vi "lab2_usrp_packet_transceiver2.vi"() -> ()   [LabVIEW 2014]
uses:
  <vilib>/addons/Modulation/Digital/General/MT Generate Bits (Galois, PN Order).vi
  <vilib>/addons/Modulation/Analog/support/mod_Set Error Source.vi
  <vilib>/addons/Modulation/Digital/Support/Common/Validators/mod_Generate Bits Validate.vi
  var_stop.vi
  <vilib>/addons/Modulation/Digital/Support/Common/Validators/mod_Generate Filter Coefficients Validate.vi
  <vilib>/addons/Modulation/Digital/General/subVIs/mod_Generate Filter Coefficients.vi
  <vilib>/measure/maspectr.llb/FFT Power Spectrum and PSD for 1 Chan (CDB).vi
  <vilib>/addons/Modulation/Digital/General/MT Apply Matched Filter (Generic).vi
  <vilib>/addons/Modulation/Digital/General/MT Align to Ideal Symbols (Generic).vi
  <instrlib>/niUSRP/niUSRP Fetch Rx Data (CDB Cluster).vi
  <instrlib>/niUSRP/niUSRP Write Tx Data (CDB Cluster).vi
  <vilib>/addons/Modulation/Digital/General/subVIs/mod_Generate Bits PN Sequence.vi
  <vilib>/addons/Modulation/Digital/General/MT Apply Pulse Shaping Filter (Generic).vi
  <vilib>/addons/Modulation/niDMT.lvlib
  <vilib>/measure/NI_MAPro.lvlib
panel:
  out "ber":dbl
  out "received bits":i32
  out "error bits":i32
  in  "random bits":i8[](array[numeric])
  out "found?":bool
  out "# elements in queue":i32
  out "Spectrum monitor":cluster{"f0":dbl, "df":dbl, "magnitude":dbl[]}(graph)={"f0"=-0.49993781867926873, "df"=0.00012436264146250465, "magnitude"=[]}
  out "RX Constellation Map":cdb[](graph)
  out "valid?":bool
  in  "Gray code?":bool
  in  "Modulation":enum16{"PSK", "QAM"}(ring)=enum."QAM"
  out "Rx String":string
  out "packet len":u32
  in  "Send":bool
  in  "filter length (symbols)":i32=8
  in  "filter parameter":dbl=0.5 format="%.2f"
  in  "pulse shaping filter (none)":T1(ring)=enum."Raised Cosine"
  in  "M-PSK (4)":i32=16 caption="M-ARY"
  in  "samples per symbol (16)":i32=4
  out "packet bits length":i32
  in  "number of samples":i64=40000
  out "RX coerced gain":dbl format="%#_6f"
  out "RX coerced carrier frequency":dbl=915000000.0 format="%#_6p"
  out "RX coerced IQ rate":dbl=4000000.0 format="%#_6p"
  in  "RX active antenna":string="RX2"
  in  "RX gain":dbl format="%#_6f"
  in  "RX device names":refnum<k15>="192.168.10.2"
  out "TX coerced gain":dbl format="%#_6f"
  out "TX coerced carrier frequency":dbl=915000000.0 format="%#_6p"
  out "coerced IQ rate":dbl=4000000.0 format="%#_6p"
  in  "TX device names":refnum<k15>="192.168.10.2"
  in  "TX gain":dbl format="%#_6f"
  in  "carrier frequency":dbl=915000000.0 format="%#_6p"
  in  "IQ rate":dbl=800000.0 format="%#_6p"
  in  "stop":bool
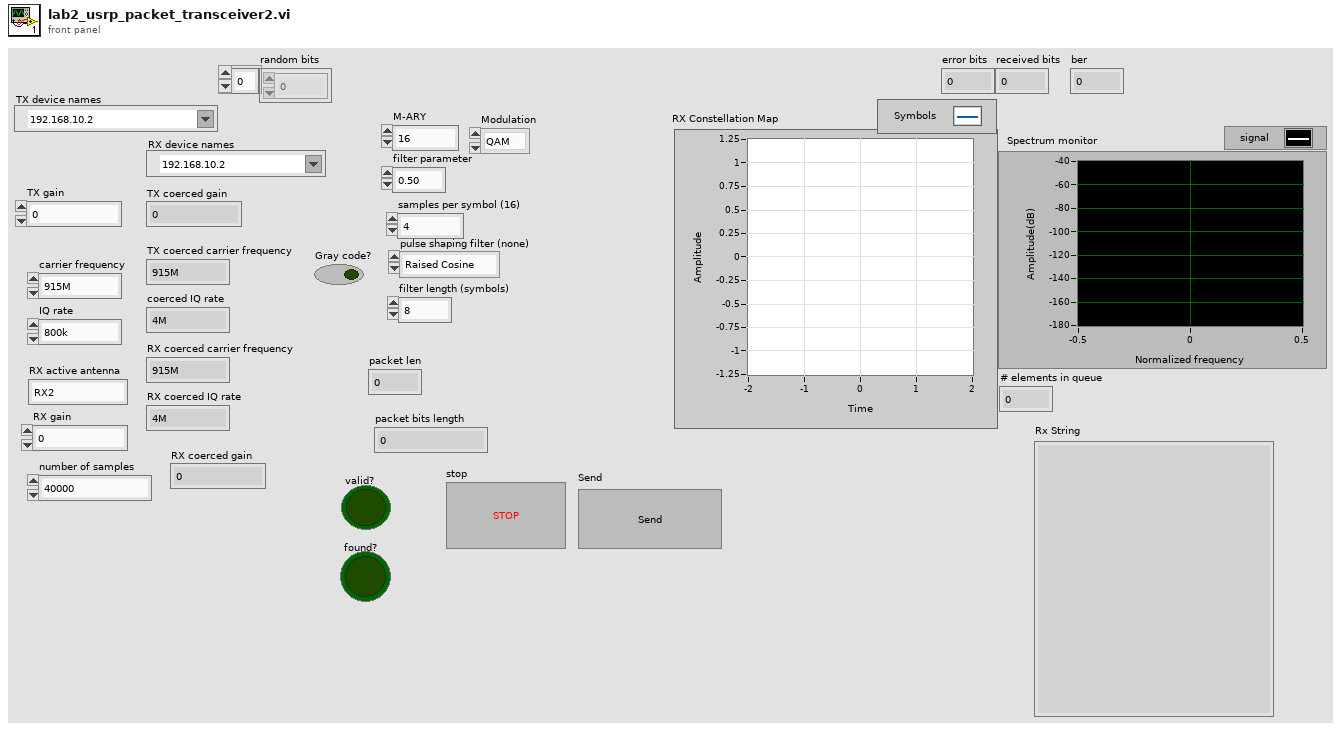
[diagram p1: front panel]
types:
  T1 = enum16{"none", "Raised Cosine", "Root Raised Cos", "Gaussian"}
  T2 = enum16{"FSK", "PSK", "QAM", "MSK", "PAM", "ASK", "CPM"}
  T3 = cluster{"samples per symbol (16)":i32, "symbol map":cdb[], "index map":u32[]}
  T4 = cluster{"samples per symbol (16)":i32, "symbol map":cdb[], i32[]}
  T5 = typedef "niAMT.lvlib/Complex Data Waveform.ctl" = cluster{"t0":dbl, "dt":dbl, "Y":cdb[]}
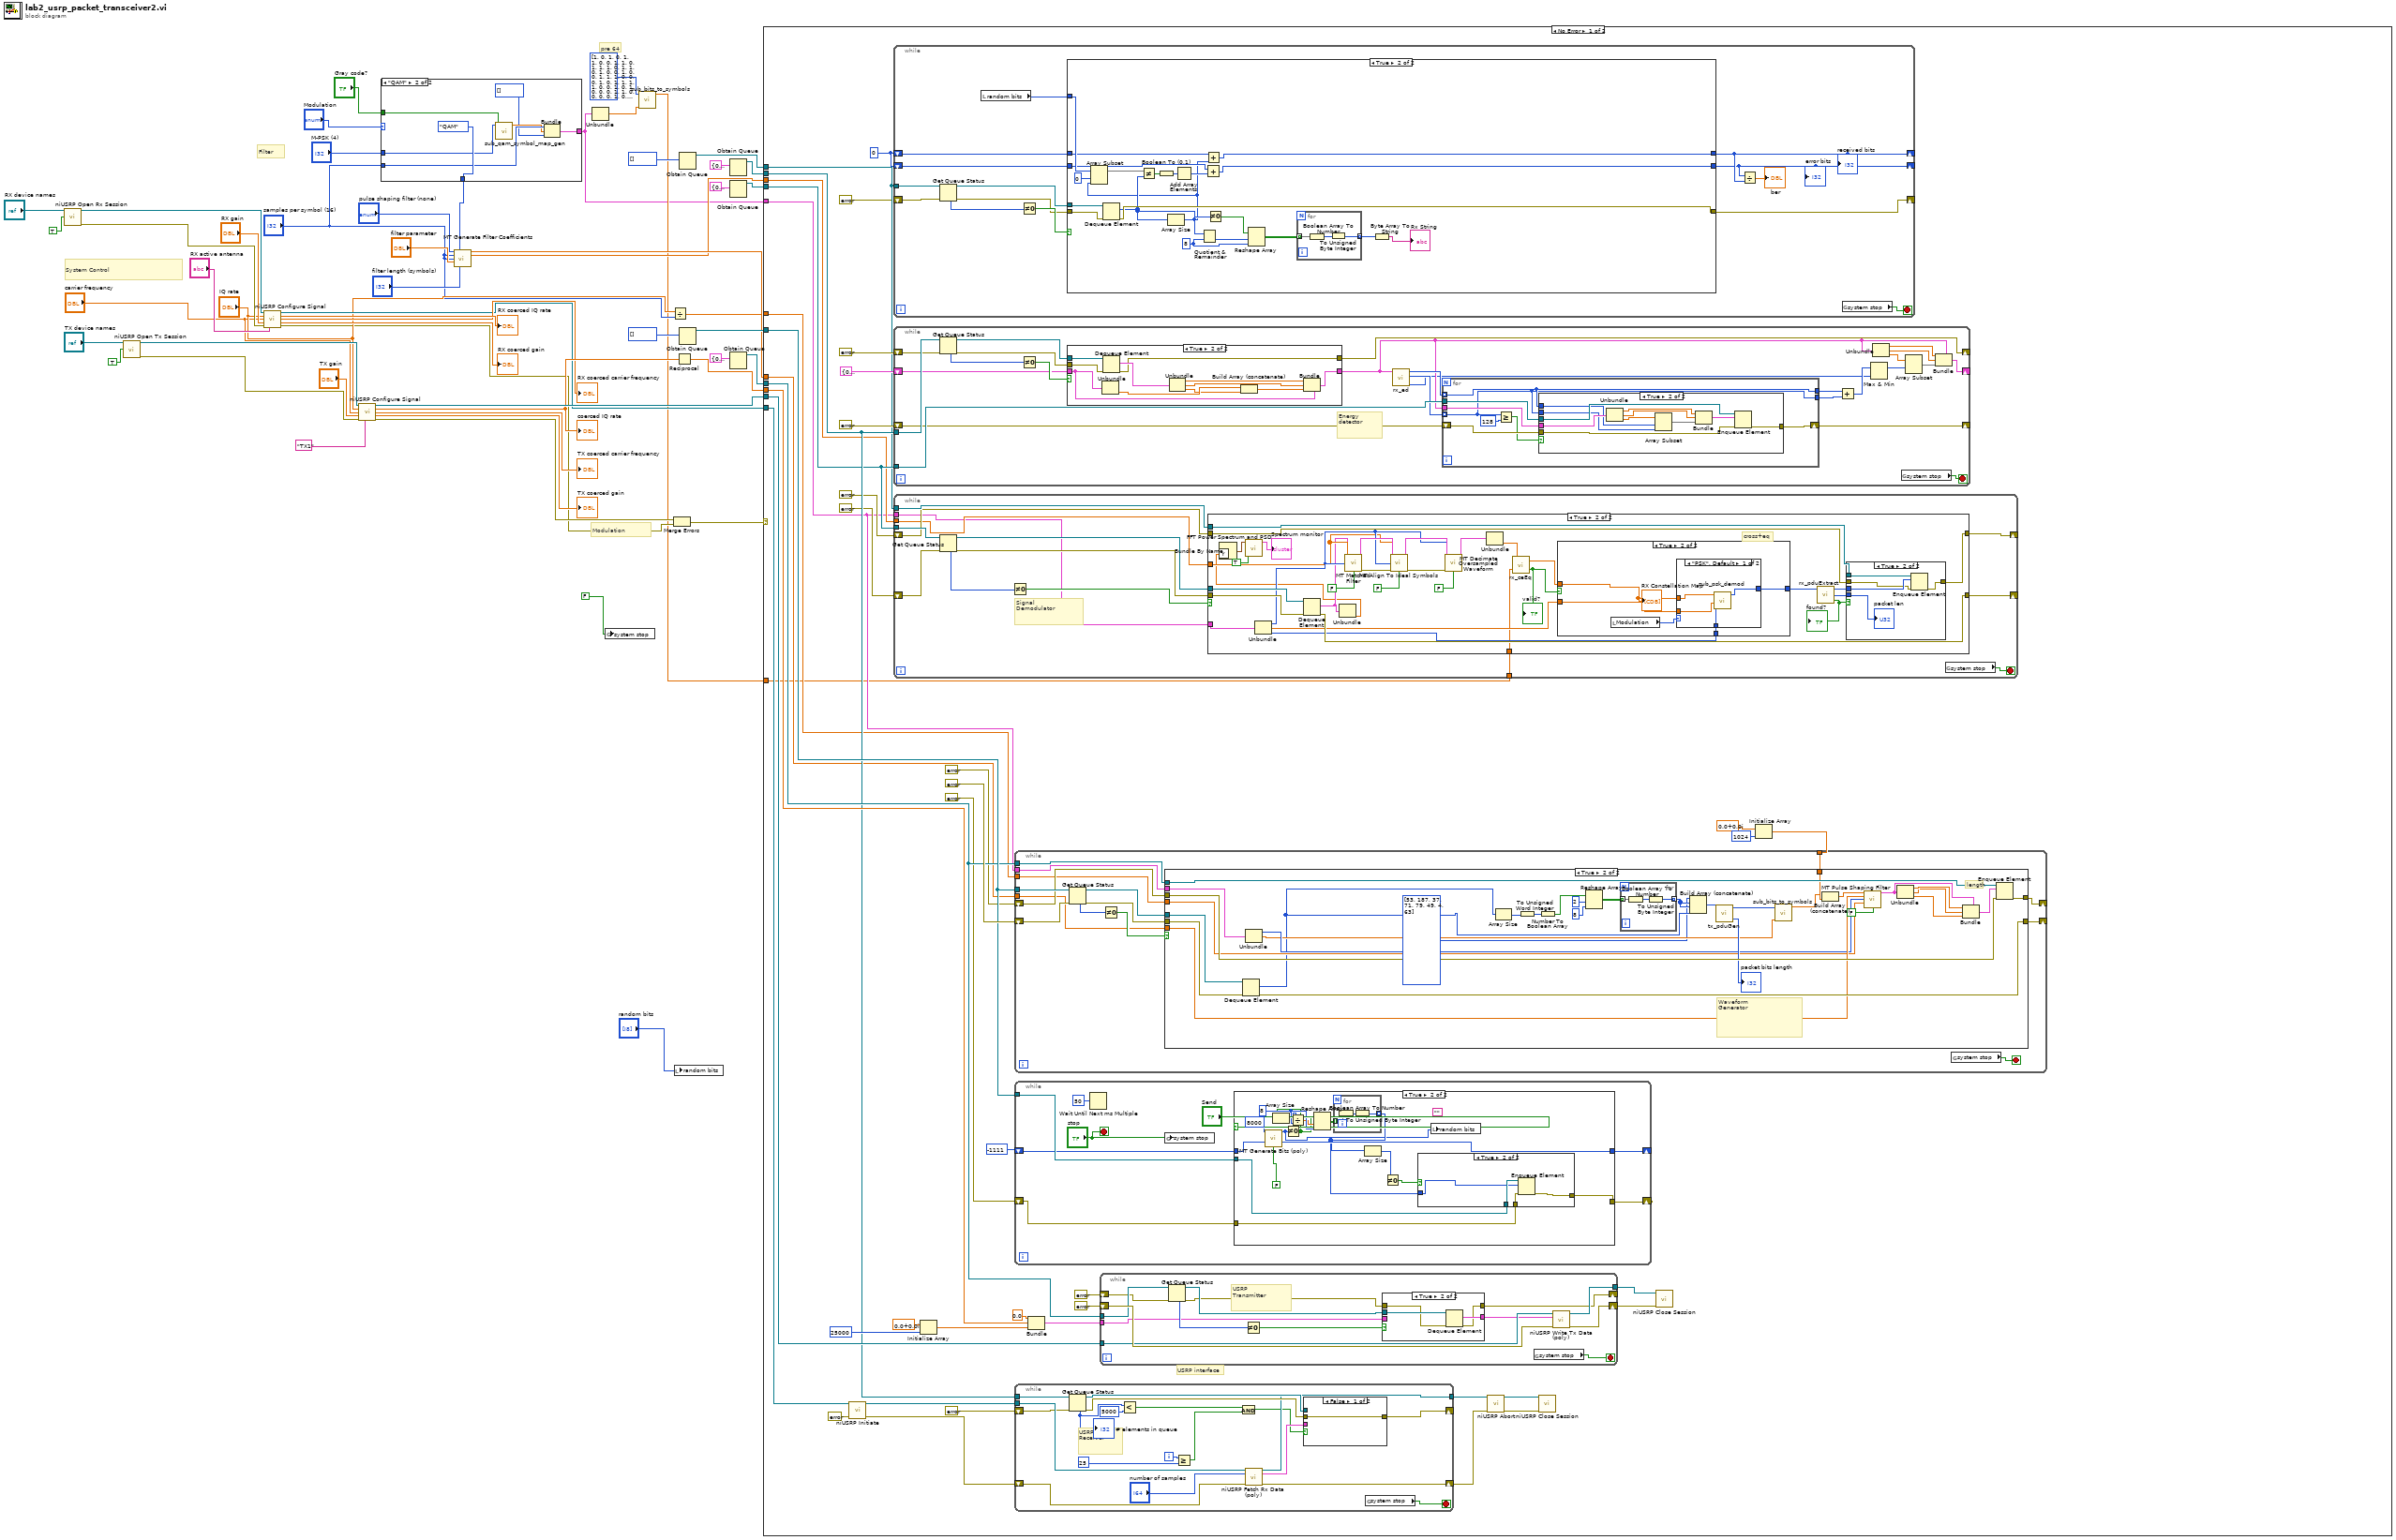
[diagram p0: block diagram]
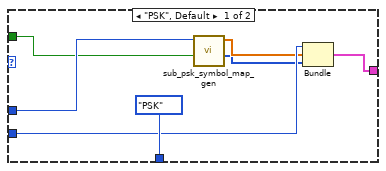
[diagram p2: hidden frame]
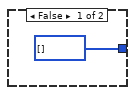
[diagram p5: hidden frame]
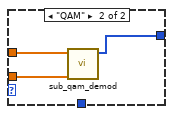
[diagram p6: hidden frame]
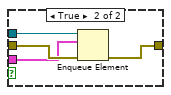
[diagram p10: hidden frame]
diagram:
  # "pre 64"
  # "Modulation"
  # "Filter"
  # "System Control"
  n1 = call <instrlib>:"niUSRP Open Rx Session.vi"("device names"="RX device names", "reset"=TRUE) -> ("session handle out"=w39:refnum<k15>, "error out"=w38:errorcluster)  [unwired: 12 in]
  n2 = call <instrlib>:"niUSRP Open Tx Session.vi"("device names"="TX device names", "reset"=TRUE) -> ("session handle out"=w52:refnum<k15>, "error out"=w51:errorcluster)  [unwired: 12 in]
  n3 = call <instrlib>:"niUSRP Configure Signal.vi"("session handle"=w39, "IQ rate"="IQ rate", "carrier frequency"="carrier frequency", "gain"="RX gain", "error in (no error)"=w38, "active antenna"="RX active antenna") -> ("session handle out"=w30:refnum<k15>, "coerced IQ rate"=→"RX coerced IQ rate":dbl, "coerced carrier frequency"=→"RX coerced carrier frequency":dbl, "coerced gain"=→"RX coerced gain":dbl, "error out"=w14:errorcluster)  [unwired: 5 in]
  n4 = call <instrlib>:"niUSRP Configure Signal.vi"("session handle"=w52, "IQ rate"="IQ rate", "carrier frequency"="carrier frequency", "gain"="TX gain", "error in (no error)"=w51, "active antenna"="TX1") -> ("session handle out"=w43:refnum<k15>, "coerced IQ rate"=w41:dbl, "coerced carrier frequency"=→"TX coerced carrier frequency":dbl, "coerced gain"=→"TX coerced gain":dbl, "error out"=w15:errorcluster)  [unwired: 5 in]
  "coerced IQ rate" <- w41
  n5 = case shown="\"QAM\"" "Modulation" {
    tunnel: [T2."PSK" ("modulation type") T2."QAM" ("modulation type")] -> w9
    tunnel: "M-PSK (4)" -> [w59 w65]
    tunnel: "Gray code?" -> [w58 w66]
    tunnel: "samples per symbol (16)" -> [w57 w64]
    tunnel: [w54 w61] -> w2
    frame "PSK", Default {
      n6 = call "sub_psk_symbol_map_gen.vi"("Gray code?"=w58, "M-PSK"=w59) -> ("index map"=w55:u32[], "symbol map"=w56:cdb[])  [unwired: 8 in]
      n7 = Bundle("samples per symbol (16)"=w57, "symbol map"=w56, "index map"=w55) -> (w54:T3)  [unwired: 1 in]
    }
    frame "QAM" {
      n8 = call "sub_qam_symbol_map_gen.vi"("Gray code?"=w66, "M-QAM"=w65) -> ("symbol map"=w63:cdb[])  [unwired: 9 in]
      n9 = Bundle("samples per symbol (16)"=w64, "symbol map"=w63, i32[] []) -> (w61:T4)  [unwired: 1 in]
    }
  }
  n10 = call <vilib>:"MT Generate Filter Coefficients.vi"("pulse shaping filter (none)"="pulse shaping filter (none)", "modulation type"=w9, "pulse shaping samples per symbol (16)"="samples per symbol (16)", "matched samples per symbol (16)"="samples per symbol (16)", "filter parameter"="filter parameter", "filter length (symbols)"="filter length (symbols)") -> ("pulse shaping filter coefficients"=w20:dbl[], "matched filter coefficients"=w18:dbl[])  [unwired: 7 in, 1 out]
  n11 = Unbundle(w2) -> ("symbol map"=w4:cdb[])  [unwired: 2 out]
  n12 = global write "var_stop.vi" "system stop"(FALSE) -> ()
  n13 = call "sub_bits_to_symbols.vi"("symbol map"=w4, "bits"=i16[] [1, 0, 1, 0, 1, 1, 0, 0, 1, 1, 0, 1, 1, 1, 0, 1, 1, 0, 1, 0, 0, 1, 0, 0, 1, 1, 1, 0, 0, 0, 1, 0, 1, 1, 1, 1, 0, 0, 1, 0, 1, 0, 0, 0, 1, 1, 0, 0, 0, 0, 1, 0, 0, 0, 0, 0, 1, 1, 1, 1, 1, 1, 0, 0] ("preamble(64) 2")) -> ("symbols"=w3:cdb[])  [unwired: 9 in]
  n14 = Divide(x="IQ rate", y="samples per symbol (16)") -> (x/y=w19:dbl)
  n15 = Merge Errors(w15, w14) -> (w13:errorcluster)
  n16 = local write "random bits"("random bits") -> ()
  n17 = Reciprocal(x=w41) -> (1/x=w40:dbl)
  n18 = Obtain Queue(element data type=i8[] [] ("output bit stream")) -> (queue out=w25:refnum<queue>)  [unwired: 4 in, 2 out]
  n19 = Obtain Queue(element data type=i16[] []) -> (queue out=w53:refnum<queue>)  [unwired: 4 in, 2 out]
  n20 = Obtain Queue(element data type=cluster{"t0":dbl, "dt":dbl, "Y":cdb[]} {"t0"=0.0, "dt"=0.0, "Y"=[]} ("data")) -> (queue out=w29:refnum<queue>)  [unwired: 4 in, 2 out]
  n21 = Obtain Queue(element data type=cluster{"t0":dbl, "dt":dbl, "Y":cdb[]} {"t0"=0.0, "dt"=0.0, "Y"=[]} ("data")) -> (queue out=w26:refnum<queue>)  [unwired: 4 in, 2 out]
  n22 = Obtain Queue(element data type=cluster{"t0":dbl, "dt":dbl, "Y":cdb[]} {"t0"=0.0, "dt"=1.0, "Y"=[]} ("data")) -> (queue out=w44:refnum<queue>)  [unwired: 4 in, 2 out]
  n23 = case shown="No Error" w13 {
    tunnel: w53 -> [w110 _]
    tunnel: w44 -> [w105 _]
    tunnel: w43 -> [w106 _]
    tunnel: w40 -> [w99 _]
    tunnel: w30 -> [w94 _]
    tunnel: w29 -> [w88 _]
    tunnel: w26 -> [w84 _]
    tunnel: w25 -> [w82 _]
    tunnel: w2 -> [w76 _]
    tunnel: w20 -> [w79 _]
    tunnel: w19 -> [w78 _]
    tunnel: w18 -> [w77 _]
    tunnel: w3 -> [w70 _]
    frame No Error {
      w69 = 0
      # "USRP interface"
      n24 = call <instrlib>:"niUSRP Initiate.vi"("session handle"=w94, "error in (no error)"=errorcluster {"status"=FALSE, "code"=0, "source"=""}) -> ("session handle out"=w93:refnum<k15>, "error out"=w92:errorcluster)  [unwired: 12 in]
      n25 = while {
        tunnel: w82 -> [w125]
        shift-right: [w118] -> _
        shift-left: errorcluster {"status"=FALSE, "code"=0, "source"=""} ("error out") -> [w124]
        shift-right: [w113] -> _
        shift-left: w69 -> [w116]
        shift-right: [w114] -> _
        shift-left: w69 -> [w115]
        stop <- w123 stop-if-true
        n26 = Get Queue Status(queue=w125, error in (no error)=w124) -> (queue out=w120:refnum<queue>, error out=w119:errorcluster, # elements in queue=w122:i32)  [unwired: 1 in, 5 out]
        n27 = local read "random bits"() -> (w117:i8[])
        n28 = Not Equal To 0?(x=w122) -> (x != 0?=w121:bool)
        n29 = case shown="True" w121 {
          tunnel: w120 -> [_ w149]
          tunnel: w119 -> [w128 w148]
          tunnel: [w128 w143] -> w118
          tunnel: w117 -> [_ w140]
          tunnel: w116 -> [w127 w135]
          tunnel: [w127 w134] -> w113
          tunnel: [w126 w132] -> w114
          tunnel: w115 -> [w126 w133]
          frame False {
          }
          frame True {
            w146 = 8 ("y")
            n30 = Dequeue Element(queue=w149, error in (no error)=w148) -> (element=w139:i8[], error out=w143:errorcluster)  [unwired: 1 in, 2 out]
            n31 = Array Size(array=w139) -> (size(s)=w130:i32)
            n32 = Array Subset(array=w140, index=0, length=w130) -> (w131:i8[])
            n33 = Not Equal?(x=w131, y=w139) -> (x != y?=w138:bool[])
            n34 = Boolean To (0,1)(Boolean=w138) -> (0, 1=w137:i16[])
            n35 = Add Array Elements(numeric array=w137) -> (sum=w136:i16)
            n36 = Quotient & Remainder(x=w130, y=w146) -> (floor(x/y)=w145:i32)  [unwired: 1 out]
            n37 = Add(x=w135, y=w136) -> (x+y=w134:i32)
            n38 = Add(x=w133, y=w130) -> (x+y=w132:i32)
            n39 = Not Equal To 0?(x=w139) -> (x != 0?=w147:bool[])
            n40 = Reshape Array(w147, w145, w146) -> (w144:bool[][])
            n41 = for {
              tunnel: w144 -> [w152] mode=indexing
              tunnel: [w151] -> w142 mode=indexing
              n42 = Boolean Array To Number(Boolean array=w152) -> (number=w150:u32)
              n43 = To Unsigned Byte Integer(number=w150) -> (unsigned 8bit integer=w151:u8)
            }
            n44 = Byte Array To String(unsigned byte array=w142) -> (string=→"Rx String":string)
          }
        }
        "error bits" <- w113
        "received bits" <- w114
        n45 = Divide(x=w113, y=w114) -> (x/y=→"ber":dbl)
        n46 = global read "var_stop.vi" "system stop"() -> (w123:bool)
      }
      n47 = while {
        tunnel: w88 -> [w244]
        shift-right: [w237] -> _
        shift-left: errorcluster {"status"=FALSE, "code"=0, "source"=""} ("error out") -> [w243]
        shift-right: [w223] -> _
        shift-left: cluster{"t0":dbl, "dt":dbl, "Y":cdb[]} {"t0"=0.0, "dt"=0.0, "Y"=[]} ("data") -> [w238]
        tunnel: w84 -> [w236]
        shift-right: [w235] -> _
        shift-left: errorcluster {"status"=FALSE, "code"=0, "source"=""} ("error out") -> [w234]
        stop <- w233 stop-if-true
        # "Energy\ndetector"
        n48 = Get Queue Status(queue=w244, error in (no error)=w243) -> (queue out=w239:refnum<queue>, error out=w240:errorcluster, # elements in queue=w242:i32)  [unwired: 1 in, 5 out]
        n49 = Not Equal To 0?(x=w242) -> (x != 0?=w241:bool)
        n50 = case shown="True" w241 {
          tunnel: w240 -> [w266 w277]
          tunnel: w239 -> [_ w276]
          tunnel: w238 -> [w265 w271]
          tunnel: [w266 w268] -> w237
          tunnel: [w265 w267] -> w230
          frame False {
          }
          frame True {
            n51 = Unbundle(w271) -> ("Y"=w274:cdb[])  [unwired: 2 out]
            n52 = Dequeue Element(queue=w276, error in (no error)=w277) -> (element=w275:cluster{"t0":dbl, "dt":dbl, "Y":cdb[]}, error out=w268:errorcluster)  [unwired: 1 in, 2 out]
            n53 = Unbundle(w275) -> ("t0"=w270:dbl, "dt"=w269:dbl, "Y"=w273:cdb[])
            n54 = Build Array (concatenate)(w274, w273) -> (w272:cdb[])
            n55 = Bundle(cluster=w271, "t0"=w270, "dt"=w269, "Y"=w272) -> (w267:cluster{"t0":dbl, "dt":dbl, "Y":cdb[]})
          }
        }
        n56 = call "rx_ed.vi"("Wavefrom"=w230) -> ("first pulse"=w220:i32, "length"=w231:i32[], "start index"=w232:i32[])  [unwired: 8 in]
        n57 = for {
          tunnel: w236 -> [w252]
          tunnel: w230 -> [w249]
          shift-right: [w251] -> w235
          shift-left: w234 -> [w250]
          tunnel: w232 -> [w248] mode=indexing
          tunnel: w231 -> [w247] mode=indexing
          tunnel: [w248] -> w226
          tunnel: [w247] -> w225
          n58 = Greater Or Equal?(x=w247, y=128) -> (x >= y?=w245:bool)
          n59 = case shown="True" w245 {
            tunnel: w252 -> [_ w264]
            tunnel: [w253 w263] -> w251
            tunnel: w250 -> [w253 w262]
            tunnel: w249 -> [_ w261]
            tunnel: w248 -> [_ w255]
            tunnel: w247 -> [_ w254]
            frame False {
            }
            frame True {
              n60 = Unbundle(w261) -> ("t0"=w259:dbl, "dt"=w260:dbl, "Y"=w257:cdb[])
              n61 = Array Subset(array=w257, index=w255, length=w254) -> (w256:cdb[])
              n62 = Bundle("t0"=w259, "dt"=w260, w256) -> (w258:cluster{"t0":dbl, "dt":dbl, cdb[]})  [unwired: 1 in]
              n63 = Enqueue Element(queue=w264, element=w258, error in (no error)=w262) -> (error out=w263:errorcluster)  [unwired: 1 in, 2 out]
            }
          }
        }
        n64 = Add(x=w226, y=w225) -> (x+y=w222:i32)
        n65 = Max & Min(x=w222, y=w220) -> (max(x,y)=w221:i32)  [unwired: 1 out]
        n66 = Unbundle(w230) -> ("t0"=w229:dbl, "dt"=w228:dbl, "Y"=w227:cdb[])
        n67 = global read "var_stop.vi" "system stop"() -> (w233:bool)
        n68 = Array Subset(array=w227, index=w221) -> (w224:cdb[])  [unwired: 1 in]
        n69 = Bundle(cluster=w230, "t0"=w229, "dt"=w228, "Y"=w224) -> (w223:cluster{"t0":dbl, "dt":dbl, "Y":cdb[]})
      }
      n70 = while {
        tunnel: w84 -> [w166]
        shift-right: [w160] -> _
        shift-left: errorcluster {"status"=FALSE, "code"=0, "source"=""} ("error out") -> [w165]
        tunnel: w82 -> [w159]
        shift-right: [w158] -> _
        shift-left: errorcluster {"status"=FALSE, "code"=0, "source"=""} ("error out") -> [w157]
        tunnel: w77 -> [w155]
        tunnel: w76 -> [w154]
        tunnel: w70 -> [w153]
        stop <- w156 stop-if-true
        # "Signal \nDemodulator"
        n71 = Get Queue Status(queue=w166, error in (no error)=w165) -> (queue out=w162:refnum<queue>, error out=w161:errorcluster, # elements in queue=w164:i32)  [unwired: 1 in, 5 out]
        n72 = Not Equal To 0?(x=w164) -> (x != 0?=w163:bool)
        n73 = case shown="True" w163 {
          tunnel: w162 -> [_ w199]
          tunnel: w161 -> [w168 w200]
          tunnel: [w168 w198] -> w160
          tunnel: w159 -> [_ w188]
          tunnel: [w167 w187] -> w158
          tunnel: w157 -> [w167 w186]
          tunnel: w155 -> [_ w175]
          tunnel: w154 -> [_ w179]
          tunnel: w153 -> [_ w171]
          frame False {
          }
          frame True {
            # "cross+eq"
            n74 = Unbundle(w179) -> ("samples per symbol (16)"=w178:i32, "symbol map"=w177:cdb[], "index map"=w176:u32[])
            n75 = Dequeue Element(queue=w199, error in (no error)=w200) -> (element=w170:cluster{"t0":dbl, "dt":dbl, "Y":cdb[]}, error out=w198:errorcluster)  [unwired: 1 in, 2 out]
            n76 = Unbundle(w170) -> ("Y"=w169:cdb[])  [unwired: 2 out]
            n77 = Bundle By Name("Y"=w169) -> (w174:waveform(cdb))  [unwired: 1 in]
            n78 = call-poly <vilib>:"FFT Power Spectrum and PSD.vi"("dB On (F)"=TRUE, "time signal"=w174) -> ("Power Spectrum / PSD"=→"Spectrum monitor":cluster{"f0":dbl, "df":dbl, "magnitude":dbl[]})  [unwired: 6 in, 3 out]
            n79 = call-poly <vilib>:"MT Matched Filter.vi"("input complex waveform"=w170, "matched filter coefficients"=w175, "samples per symbol (16)"=w178, "reset? (T)"=FALSE) -> ("output complex waveform"=w197:T5, "error out"=w196:errorcluster)  [unwired: 10 in]
            n80 = call-poly <vilib>:"MT Align To Ideal Symbols.vi"("input complex waveform"=w197, "matched filter coefficients"=w175, "samples per symbol (16)"=w178, "error in (no error)"=w196, "reset? (T)"=FALSE) -> ("output complex waveform"=w194:T5, "error out"=w195:errorcluster)  [unwired: 8 in, 1 out]
            n81 = call <vilib>:"MT Decimate Oversampled Waveform.vi"("input complex waveform"=w194, "decimation factor"=w178, "error in (no error)"=w195, "reset? (T)"=FALSE) -> ("output complex waveform"=w193:T5)  [unwired: 10 in, 1 out]
            n82 = Unbundle(w193) -> ("Y"=w189:cdb[])  [unwired: 2 out]
            n83 = call "rx_ceEq.vi"("preamble"=w171, "symbols"=w189) -> ("valid?"=w184:bool, "eq symbols"=w185:cdb[])
            "valid?" <- w184
            n84 = case shown="True" w184 {
              tunnel: [i8[] [] ("output bit stream") w204] -> w192
              tunnel: w177 -> [_ w205]
              tunnel: w185 -> [_ w202]
              tunnel: w176 -> [_ w203]
              frame False {
              }
              frame True {
                n85 = local read "Modulation"() -> (w206:enum16{"PSK", "QAM"})
                n86 = case shown="\"PSK\", Default" w206 {
                  tunnel: w202 -> [w210 w213]
                  tunnel: w205 -> [w209 w212]
                  tunnel: [w207 w211] -> w204
                  tunnel: w203 -> [w208 _]
                  frame "PSK", Default {
                    n87 = call "sub_psk_demod.vi"("index map"=w208, "symbol map"=w209, "symbol"=w210) -> ("bitstream"=w207:i16[])  [unwired: 8 in]
                  }
                  frame "QAM" {
                    n88 = call "sub_qam_demod.vi"("symbol map"=w212, "symbol"=w213) -> ("bitstream"=w211:i16[])  [unwired: 9 in]
                  }
                }
                "RX Constellation Map" <- w202
              }
            }
            n89 = call "rx_pduExtract.vi"("output bit stream"=w192) -> ("found?"=w191:bool, "packet len"=w183:u32, "ppdu"=w190:i8[])  [unwired: 2 in]
            "found?" <- w191
            n90 = case shown="True" w191 {
              tunnel: w190 -> [_ w217]
              tunnel: w188 -> [_ w219]
              tunnel: [w214 w218] -> w187
              tunnel: w186 -> [w214 w215]
              tunnel: w183 -> [_ w216]
              frame False {
              }
              frame True {
                n91 = Enqueue Element(queue=w219, element=w217, error in (no error)=w215) -> (error out=w218:errorcluster)  [unwired: 1 in, 2 out]
                "packet len" <- w216
              }
            }
          }
        }
        n92 = global read "var_stop.vi" "system stop"() -> (w156:bool)
      }
      n93 = Initialize Array(cdb 0.0+0.0i, 25000 ("dimension size")) -> (w100:cdb[])
      n94 = while {
        tunnel: w110 -> [w379]
        shift-right: [w377] -> _
        shift-left: errorcluster {"status"=FALSE, "code"=0, "source"=""} ("error out") -> [w378]
        shift-right: [w374] -> _
        shift-left: -1111 -> [w375]
        stop <- "stop" stop-if-true
        n95 = Wait Until Next ms Multiple(millisecond multiple=u32 50) -> ()  [unwired: 1 out]
        n96 = global write "var_stop.vi" "system stop"("stop") -> ()
        n97 = case shown="True" "Send" {
          tunnel: w379 -> [_ w398]
          tunnel: w378 -> [w383 w397]
          tunnel: [w383 w396] -> w377
          tunnel: w375 -> [w382 w393]
          tunnel: [w382 w392] -> w374
          frame False {
          }
          frame True {
            w390 = 8
            (unwired) ""
            n98 = call-poly <vilib>:"MT Generate Bits (poly).vi"("total bits (128)"=8000, "seed in (0xD6BF7DF2)"=w393, "reset? (T)"=FALSE) -> ("output bit stream"=w384:i8[], "seed out"=w392:i32)  [unwired: 10 in, 1 out]
            n99 = Not Equal To 0?(x=w384) -> (x != 0?=w385:bool[])
            n100 = Array Size(array=w385) -> (size(s)=w389:i32)
            n101 = Divide(x=w389, y=w390) -> (x/y=w388:dbl)
            n102 = Reshape Array(w385, w388, w390) -> (w387:bool[][])
            n103 = for {
              tunnel: w387 -> [w402] mode=indexing
              tunnel: [w400] -> w386 mode=indexing
              n104 = Boolean Array To Number(Boolean array=w402) -> (number=w401:u32)
              n105 = To Unsigned Byte Integer(number=w401) -> (unsigned 8bit integer=w400:u8)
            }
            n106 = Array Size(array=w386) -> (size(s)=w395:i32)
            n107 = Not Equal To 0?(x=w395) -> (x != 0?=w399:bool)
            n108 = case shown="True" w399 {
              tunnel: w386 -> [_ w404]
              tunnel: w398 -> [_ w407]
              tunnel: w397 -> [w403 w406]
              tunnel: [w403 w405] -> w396
              frame False {
              }
              frame True {
                n109 = Enqueue Element(queue=w407, element=w404, error in (no error)=w406) -> (error out=w405:errorcluster)  [unwired: 1 in, 2 out]
              }
            }
            n110 = local write "random bits"(w384) -> ()
          }
        }
      }
      n111 = while {
        tunnel: w93 -> [w296]
        shift-right: [w284] -> w89
        shift-left: w92 -> [w295]
        tunnel: w88 -> [w293]
        shift-right: [w287] -> _
        shift-left: errorcluster {"status"=FALSE, "code"=0, "source"=""} ("error out") -> [w292]
        tunnel: [w285] -> w90
        i -> [w282]
        stop <- w283 stop-if-true
        # "USRP\nReceiver"
        n112 = Get Queue Status(queue=w293, error in (no error)=w292) -> (queue out=w289:refnum<queue>, error out=w288:errorcluster, # elements in queue=w291:i32)  [unwired: 1 in, 5 out]
        "# elements in queue" <- w291
        n113 = Less?(x=w291, y=5000) -> (x < y?=w280:bool)
        n114 = Greater Or Equal?(x=w282, y=25) -> (x >= y?=w279:bool)
        n115 = And(x=w280, y=w279) -> (x .and. y?=w278:bool)
        n116 = call-poly <instrlib>:"niUSRP Fetch Rx Data (poly).vi"("session handle"=w296, "number of samples"="number of samples", "error in (no error)"=w295) -> ("session handle out"=w285:refnum<k15>, "data"=w286:cluster{"t0":dbl, "dt":dbl, "Y":cdb[]}, "error out"=w284:errorcluster)  [unwired: 9 in, 1 out]
        n117 = case shown="False" w278 {
          tunnel: w289 -> [_ w301]
          tunnel: w288 -> [w297 w300]
          tunnel: [w297 w299] -> w287
          tunnel: w286 -> [_ w298]
          frame False {
          }
          frame True {
            n118 = Enqueue Element(queue=w301, element=w298, error in (no error)=w300) -> (error out=w299:errorcluster)  [unwired: 1 in, 2 out]
          }
        }
        n119 = global read "var_stop.vi" "system stop"() -> (w283:bool)
      }
      n120 = Bundle(0.0, w99, w100) -> (w97:cluster{dbl, dbl, cdb[]})  [unwired: 1 in]
      n121 = while {
        shift-right: [w311] -> w109
        shift-left: errorcluster {"status"=FALSE, "code"=0, "source"=""} ("error out") -> [w309]
        tunnel: [w310] -> w108
        tunnel: w106 -> [w308]
        tunnel: w105 -> [w306]
        shift-right: [w304] -> _
        shift-left: errorcluster {"status"=FALSE, "code"=0, "source"=""} ("error out") -> [w305]
        tunnel: w97 -> [w303]
        stop <- w302 stop-if-true
        # "USRP\nTransmitter"
        n122 = Get Queue Status(queue=w306, error in (no error)=w305) -> (queue out=w313:refnum<queue>, error out=w312:errorcluster, # elements in queue=w315:i32)  [unwired: 1 in, 5 out]
        n123 = Not Equal To 0?(x=w315) -> (x != 0?=w314:bool)
        n124 = case shown="True" w314 {
          tunnel: w313 -> [_ w321]
          tunnel: w312 -> [w316 w320]
          tunnel: [w317 w319] -> w307
          tunnel: [w316 w318] -> w304
          tunnel: w303 -> [w317 _]
          frame False {
          }
          frame True {
            n125 = Dequeue Element(queue=w321, error in (no error)=w320) -> (element=w319:cluster{"t0":dbl, "dt":dbl, "Y":cdb[]}, error out=w318:errorcluster)  [unwired: 1 in, 2 out]
          }
        }
        n126 = global read "var_stop.vi" "system stop"() -> (w302:bool)
        n127 = call-poly <instrlib>:"niUSRP Write Tx Data (poly).vi"("session handle"=w308, "data"=w307, "error in (no error)"=w309) -> ("session handle out"=w310:refnum<k15>, "error out"=w311:errorcluster)  [unwired: 11 in]
      }
      n128 = call <instrlib>:"niUSRP Abort.vi"("session handle"=w90, "error in (no error)"=w89) -> ("session handle out"=w96:refnum<k15>, "error out"=w95:errorcluster)  [unwired: 12 in]
      n129 = call <instrlib>:"niUSRP Close Session.vi"("session handle"=w96, "error in (no error)"=w95) -> ()  [unwired: 13 in, 1 out]
      n130 = call <instrlib>:"niUSRP Close Session.vi"("session handle"=w108, "error in (no error)"=w109) -> ()  [unwired: 13 in, 1 out]
      n131 = Initialize Array(cdb 0.0+0.0i, 1024 ("dimension size")) -> (w71:cdb[])
      n132 = while {
        tunnel: w110 -> [w333]
        shift-right: [w330] -> _
        shift-left: errorcluster {"status"=FALSE, "code"=0, "source"=""} ("error out") -> [w336]
        tunnel: w105 -> [w329]
        shift-right: [w328] -> _
        shift-left: errorcluster {"status"=FALSE, "code"=0, "source"=""} ("error out") -> [w327]
        tunnel: w76 -> [w325]
        tunnel: w79 -> [w324]
        tunnel: w78 -> [w323]
        tunnel: w71 -> [w322]
        stop <- w326 stop-if-true
        n133 = Get Queue Status(queue=w333, error in (no error)=w336) -> (queue out=w331:refnum<queue>, error out=w332:errorcluster, # elements in queue=w335:i32)  [unwired: 1 in, 5 out]
        n134 = Not Equal To 0?(x=w335) -> (x != 0?=w334:bool)
        n135 = case shown="True" w334 {
          tunnel: w332 -> [w338 w370]
          tunnel: w331 -> [_ w369]
          tunnel: [w338 w368] -> w330
          tunnel: w329 -> [_ w363]
          tunnel: [w337 w362] -> w328
          tunnel: w327 -> [w337 w361]
          tunnel: w325 -> [_ w358]
          tunnel: w324 -> [_ w357]
          tunnel: w323 -> [_ w356]
          tunnel: w322 -> [_ w346]
          frame False {
          }
          frame True {
            # "length"
            # "Waveform \nGenerator"
            n136 = Dequeue Element(queue=w369, error in (no error)=w370) -> (element=w342:i16[], error out=w368:errorcluster)  [unwired: 1 in, 2 out]
            n137 = Unbundle(w358) -> ("samples per symbol (16)"=w352:i32, "symbol map"=w344:cdb[])  [unwired: 1 out]
            n138 = Array Size(array=w342) -> (size(s)=w354:i32)
            n139 = To Unsigned Word Integer(number=w354) -> (unsigned 16bit integer=w353:u16)
            n140 = Number To Boolean Array(number=w353) -> (Boolean array=w367:bool[])
            n141 = Reshape Array(w367, 2 ("dimension size"), 8 ("dimension size")) -> (w364:bool[][])
            n142 = for {
              tunnel: w364 -> [w373] mode=indexing
              tunnel: [w371] -> w355 mode=indexing
              n143 = Boolean Array To Number(Boolean array=w373) -> (number=w372:u32)
              n144 = To Unsigned Byte Integer(number=w372) -> (unsigned 8bit integer=w371:u8)
            }
            n145 = Build Array (concatenate)(u8[] [53, 187, 37, 71, 79, 49, 4, 63] ("Array 2"), w355, w355, w342) -> (w360:i16[])
            n146 = call "tx_pduGen.vi"("byte array"=w360) -> ("packet bits length"=→"packet bits length":i32, "pdu"=w345:i32[])  [unwired: 3 in]
            n147 = call "sub_bits_to_symbols.vi"("symbol map"=w344, "bits"=w345) -> ("symbols"=w343:cdb[])  [unwired: 9 in]
            n148 = Build Array (concatenate)(w343, w346) -> (w339:cdb[])
            n149 = call-poly <vilib>:"MT Pulse Shaping Filter.vi"("symbols"=w339, "pulse shaping filter coefficients"=w357, "samples per symbol (16)"=w352, "symbol rate (Hz)"=w356, "reset? (T)"=FALSE) -> ("output complex waveform"=w351:T5)  [unwired: 9 in, 1 out]
            n150 = Unbundle(w351) -> ("t0"=w350:dbl, "dt"=w349:dbl, "Y"=w341:cdb[])
            n151 = Bundle(cluster=w351, "t0"=w350, "dt"=w349, "Y"=w341) -> (w348:T5)
            n152 = Enqueue Element(queue=w363, element=w348, error in (no error)=w361) -> (error out=w362:errorcluster)  [unwired: 1 in, 2 out]
          }
        }
        n153 = global read "var_stop.vi" "system stop"() -> (w326:bool)
      }
    }
    frame Error {
    }
  }
